vi "Event Create.vi"(9 "Actor":refnum<class "Actor.lvclass">, 10 "Alias":string, 11 "Ex Queue Actor in":refnum<class "Ex Queue Actor.lvclass">) -> (3 "Ex Queue Actor out":refnum<class "Ex Queue Actor.lvclass">)   [LabVIEW 2021, in "Ex Queue Actor.lvlib" / "Ex Queue Actor.lvclass"]
uses:
  Actor/Actor/Actor.lvclass
  Ex Queue Actor.lvclass
  Ex Queue Actor.lvclass/Ex Queue Actor.ctl
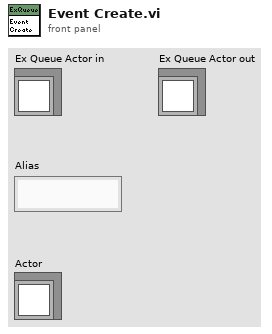
[diagram p1: front panel]
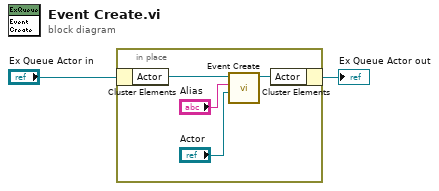
[diagram p0: block diagram]
diagram:
  n1 = in-place {
    n2 = in-place-cluster #1("Ex Queue Actor in") -> ("Actor"=w6:refnum<class "Actor.lvclass">)
    n3 = call-dynamic "Event Create.vi"("Actor"="Actor", "Alias"="Alias", "Event Create in"=w6) -> ("Event Create out"=w5:refnum<class "Actor.lvclass">)  [unwired: 8 in]
    n4 = in-place-cluster #1("Actor"=w5) -> (→"Ex Queue Actor out":refnum<class "Ex Queue Actor.lvclass">)
  }
